vi "MultiAxisControl.vi"() -> ()   [LabVIEW 2017]
uses:
  Utility/AxisControl.ctl
  Motion/AbortSingle.vi
  Motion/MoveIncSingle.vi
  Motion/FreerunSingle.vi
  Motion/EnableSingle.vi
  Motion/DisableSingle.vi
  Motion/FaultAckSingle.vi
  Motion/HomeSingle.vi
  Parameters/GetAxisParameterString.vi
  Parameters/GetAxisParameterDouble.vi
panel:
  in  "Go":bool
  out "Status":string
  in  "StopProgram":bool caption="Stop"
  out "do stop":bool
  in  "stop":bool
  out "Error":string
  in  "Init":bool=TRUE
  in  "Abort Motion":bool
  in  "Reset Controller":bool
  in  "In Task:":i32(ring)=1 items=["Auxiliary", "T1", "T2", "T3", "T4"]
  in  "ExecuteProgram":bool caption="Execute"
  in  "Program:":path
  in  "Axes":T1[](array[typedef])
  in  "Status":string
  in  "Execute":bool
  in  "Command:":string
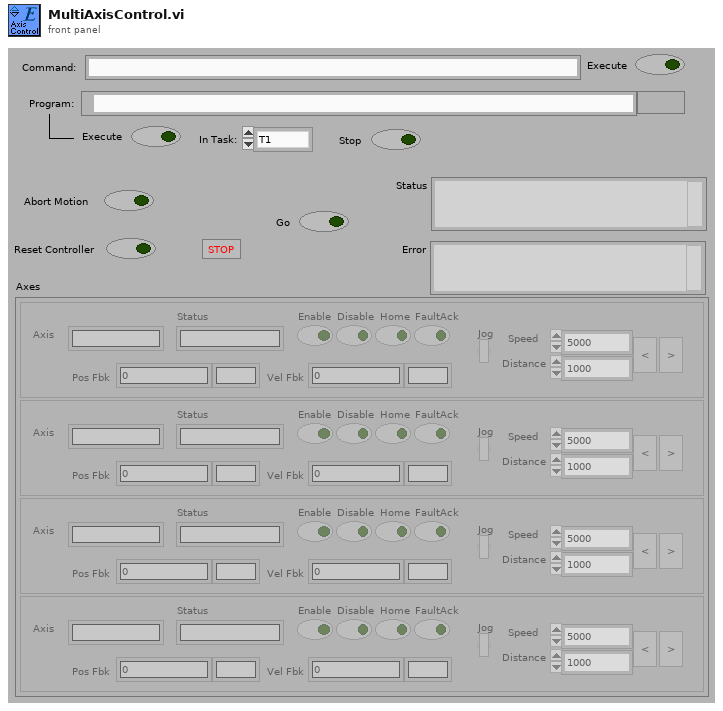
[diagram p1: front panel]
types:
  T1 = typedef "AxisControl.ctl" = cluster{"Axis":string, "Enable":bool, "Disable":bool, "Home":bool, "FaultAck":bool, "Jog":bool, "Speed":dbl, "Distance":dbl, "Jog Left":bool, "Jog Right":bool, "Status":string, "Pos Fbk":dbl, "Vel Fbk":dbl, "Pos Units":string, "Vel Units":string}
  T2 = cluster{"new reference":refnum<k24>, "Event Callback":refnum<k27>, "ControllerDiagPacket":refnum<user-event>, "Event Registration Refnum":refnum<event-registration>}
  T3 = enum32{"invalid app kind", "Development System", "Run Time System", "Student Edition", "Embedded LabVIEW", "Evaluation", "Custom"}
  T4 = cluster{"Axis":string, "Enable":bool, "Disable":bool, "Home":bool, "FaultAck":bool, "Jog":bool, "Speed":dbl, "Distance":dbl, "Jog Left":bool, "Jog Right":bool, "Status":string, "Pos Fbk":dbl, "Vel Fbk":dbl, "Pos Units":string, "Vel Units":string}
  T5 = typedef "AxisDiagPacket.ctl" = cluster{"Axis Name":string, "Acceleration Command":dbl, "Amplifier Temperature":sgl, "Analog Input 0":dbl, "Analog Input 1":dbl, "Analog Output 0":dbl, "Analog Output 1":dbl, "Axis Fault (num)":i32, "Axis Fault (str)":string, "Axis Fault (bits)":cluster{"AmplifierFault":bool, "AmplifierTemperatureFault":bool, "CcwEndOfTravelLimitFault":bool, "CcwSoftwareLimitFault":bool, "CommunicationLostFault":bool, "CwEndOfTravelLimitFault":bool, "CwSoftwareLimitFault":bool, "EmergencyStopFault":bool, "EncoderFault":bool, "ExternalFault":bool, "FeedbackScalingFault":bool, "HallSensorFault":bool, "MarkerSearchFault":bool, "MaxVelocityCommandFault":bool, "MotorTemperatureFault":bool, "None":bool, "OverCurrentFault":bool, "PositionErrorFault":bool, "PositionFeedbackFault":bool, "VelocityErrorFault":bool, "VelocityFeedbackFault":bool, "VoltageClampFault":bool, "PowerSupplyFault":bool}, "Axis Status (num)":i32, "Axis Status (str)":string, "Axis Status (bits)":cluster{"AccelerationPhase":bool, "AutofocusActive":bool, "BrakeOutput":bool, "CalibrationActive":bool, "CalibrationEnabled":bool, "CcwEndOfTravelLimitInput":bool, "CommandShapingFilterDone":bool, "CosineEncoderError":bool, "CurrentClamp":bool, "CwEndOfTravelLimitInput":bool, "DecelerationPhase":bool, "EmergencyStopInput":bool, "Enabled":bool, "GantryMasterActive":bool, "GantryModeActive":bool, "HallAInput":bool, "HallBInput":bool, "HallCInput":bool, "Homed":bool, "HomeLimitInput":bool, "Homing":bool, "InPosition":bool, "InPosition2":bool, "JoystickControl":bool, "MarkerInput":bool, "MasterMotionSuppressed":bool, "MasterSlaveControl":bool, "MotionIsCw":bool, "MoveActive":bool, "None":bool, "PositionCaptureActive":bool, "ServoControl":bool, "SineEncoderError":bool}, "Current Command":sgl, "Current Error":sgl, "Current Feedback":sgl, "Digital Input 0":i32, "Digital Input 1":i32, "Digital Input 2":i32, "Digital Output 0":i32, "Digital Output 1":i32, "Digital Output 2":i32, "Position Feedback Auxiliary":dbl, "Position Command":dbl, "Position Error":dbl, "Position Feedback":dbl, "Program Position Command":dbl, "Program Position Error":dbl, "Program Position Feedback":dbl, "Velocity Command":dbl, "Velocity Error":dbl, "Velocity Feedback":dbl}
  T6 = cluster{"Axis":string, "Enable":bool, "Disable":bool, "Home":bool, "FaultAck":bool, "Jog":bool, "Speed":dbl, "Distance":dbl, "Jog Left":bool, "Jog Right":bool, "Status":string, "Pos Fbk":dbl, "Vel Fbk":dbl, "Pos Units":string, "Vel Units":string}[]
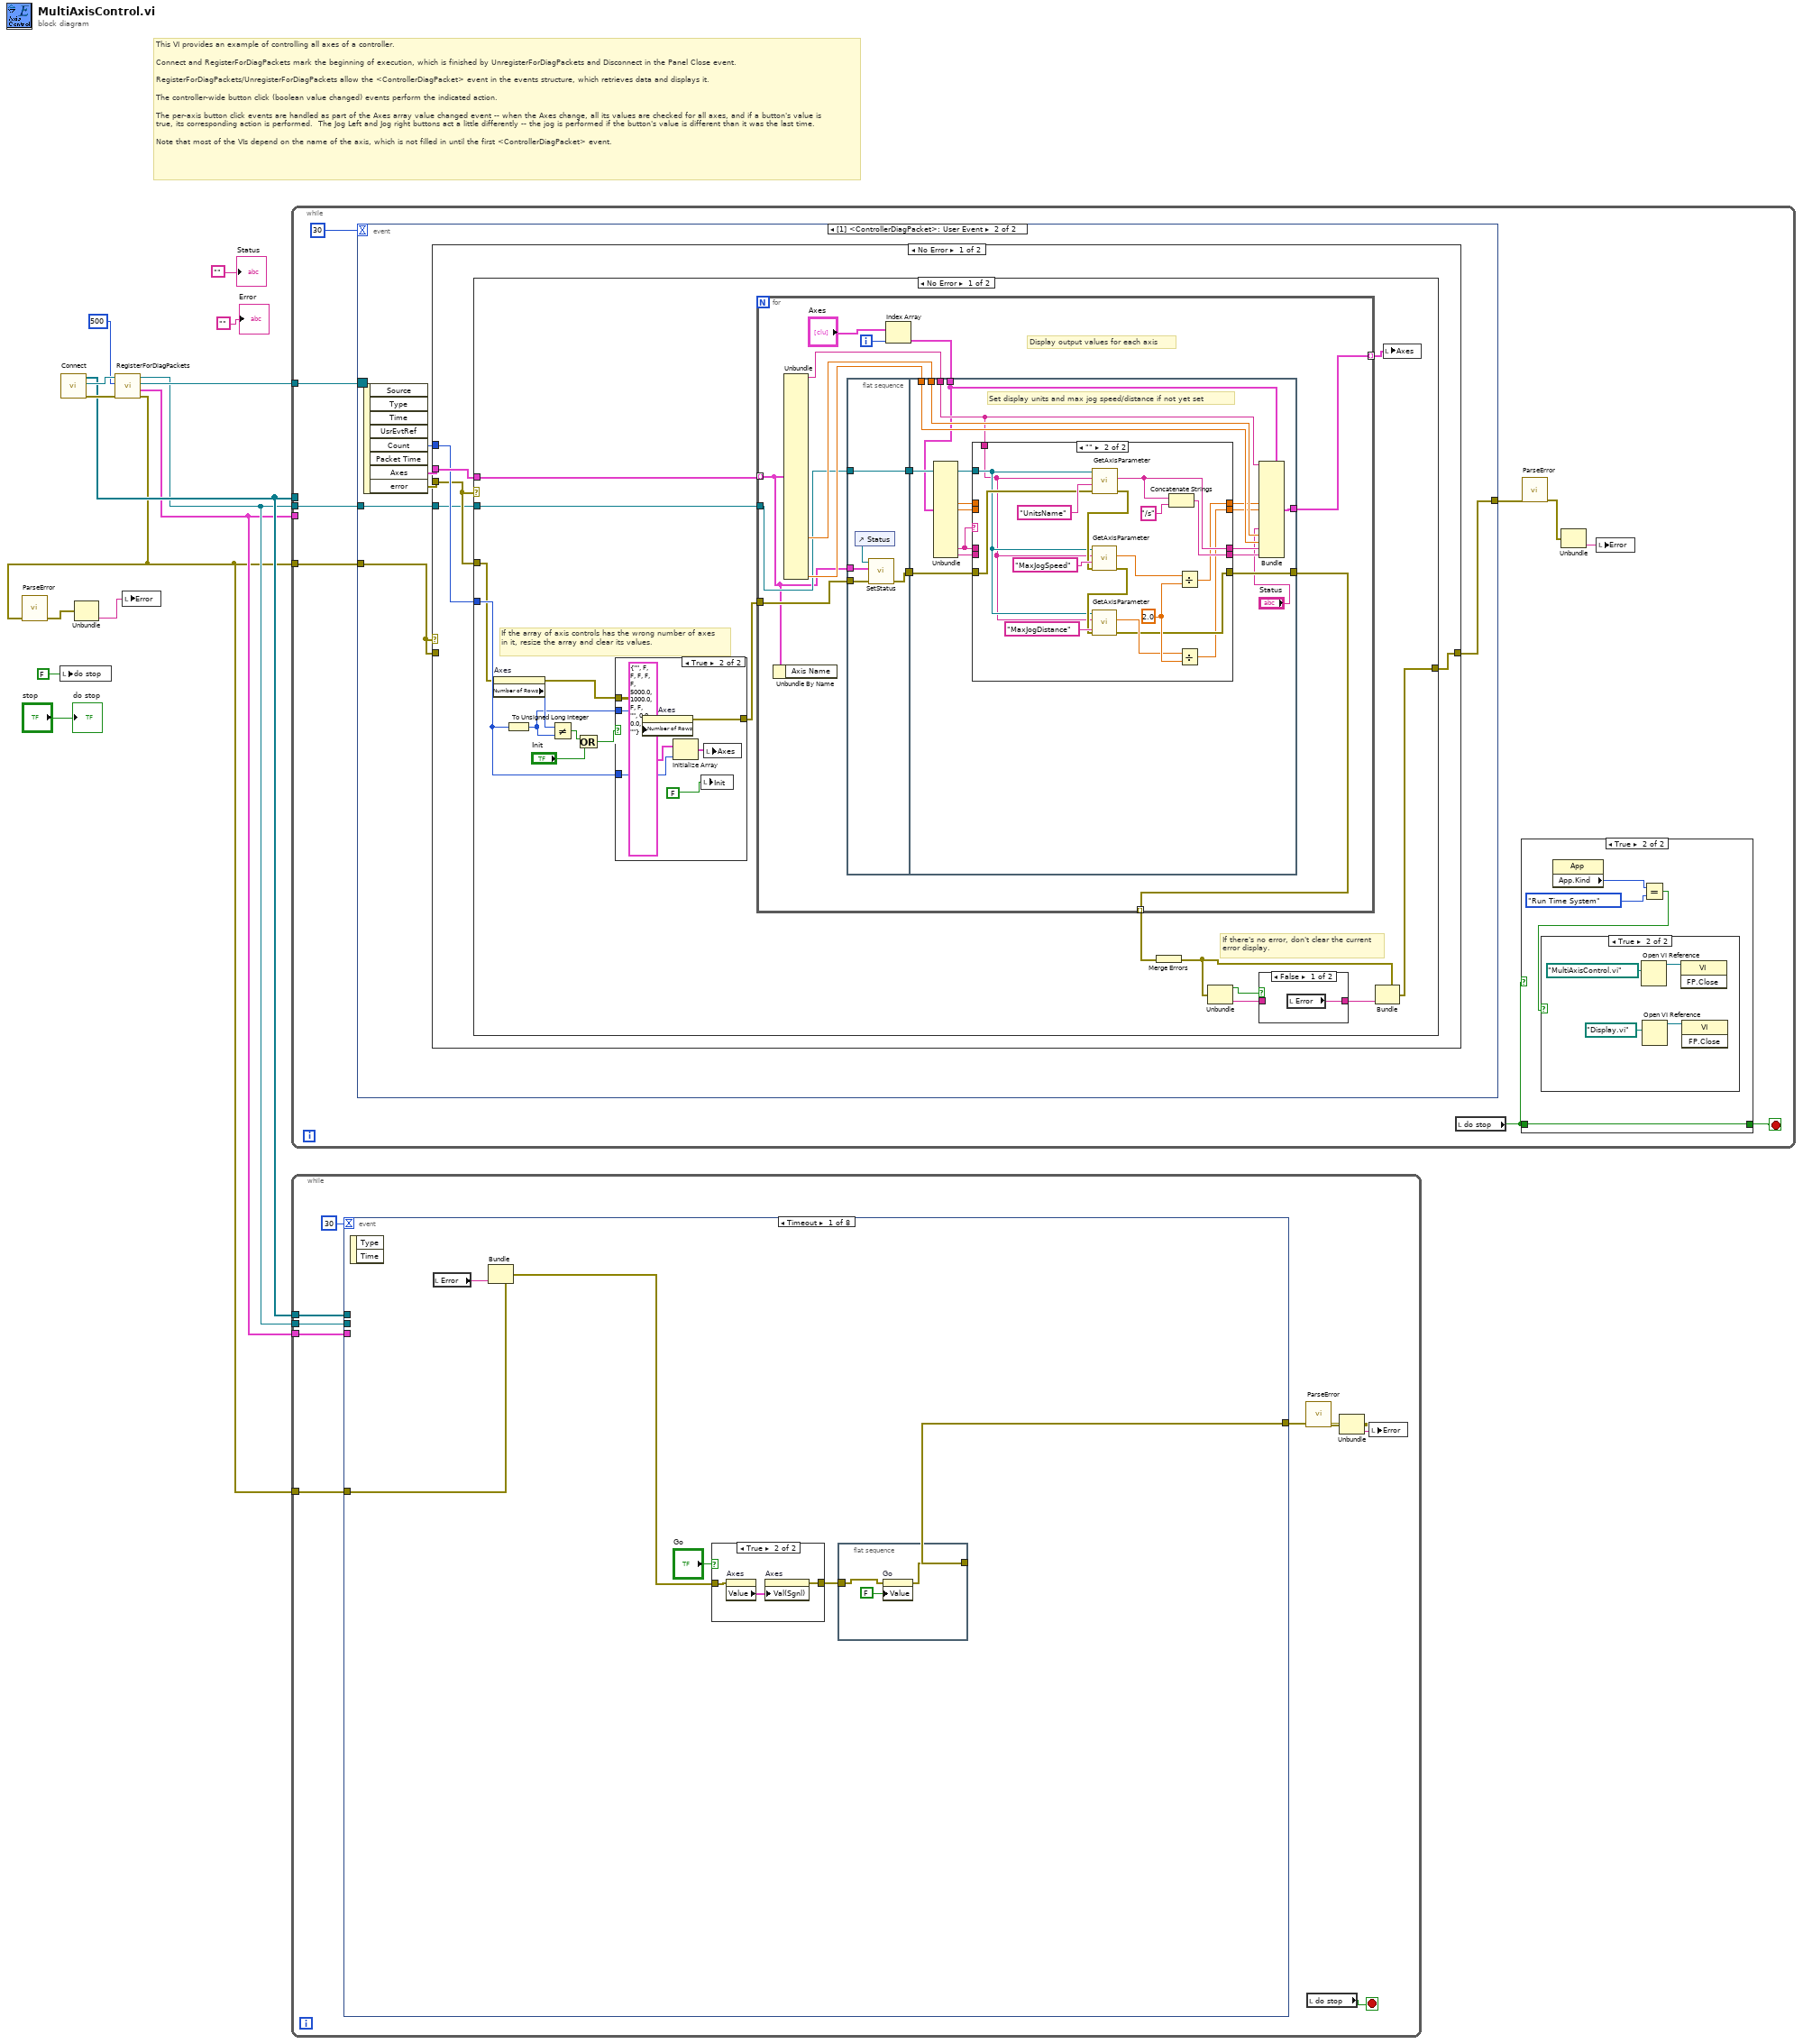
[diagram p0: block diagram]
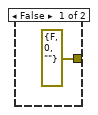
[diagram p2: hidden frame]
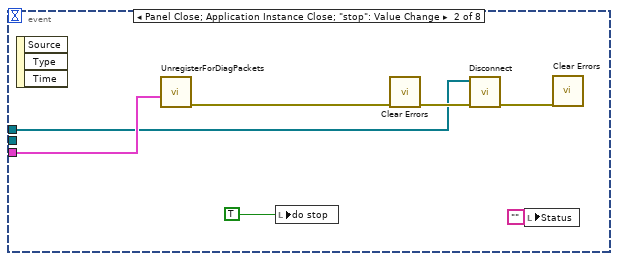
[diagram p3: hidden frame]
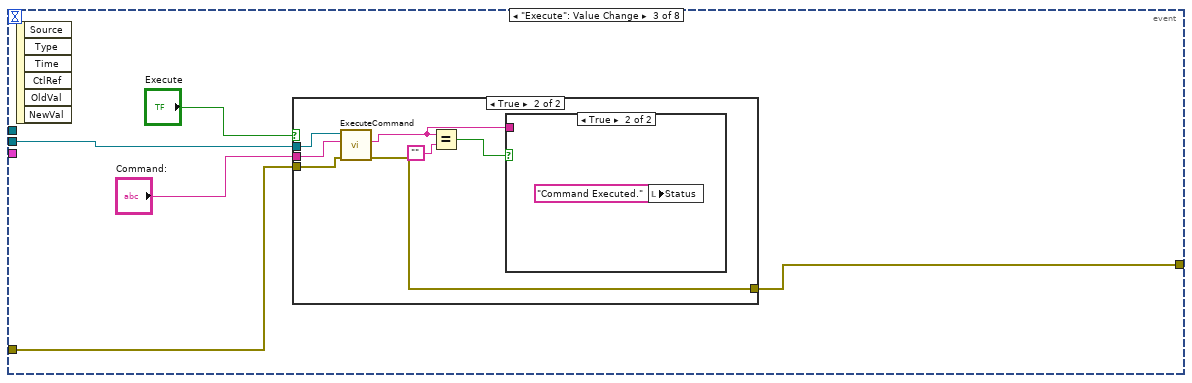
[diagram p4: hidden frame]
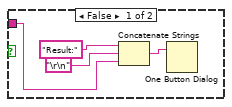
[diagram p6: hidden frame]
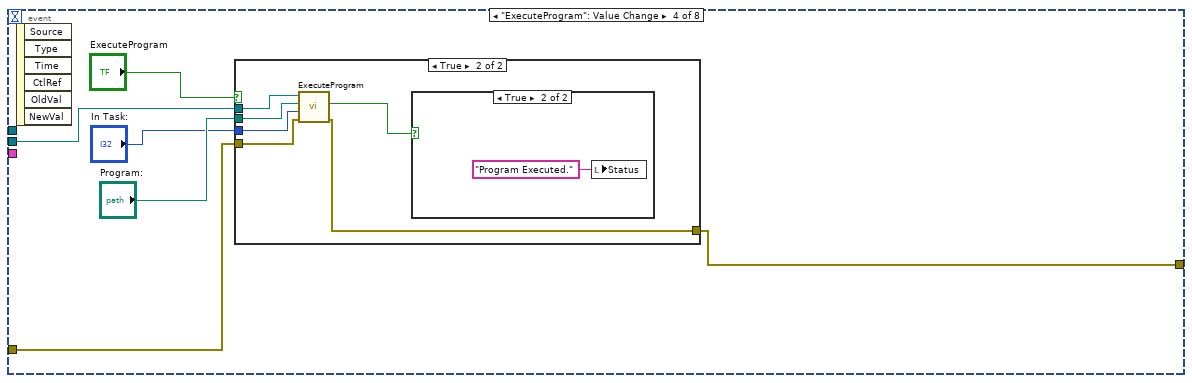
[diagram p7: hidden frame]
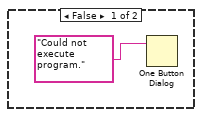
[diagram p9: hidden frame]
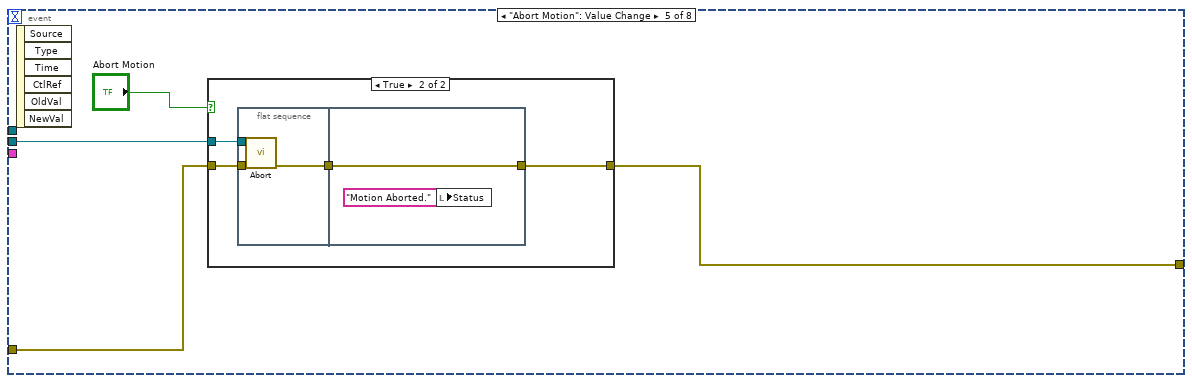
[diagram p10: hidden frame]
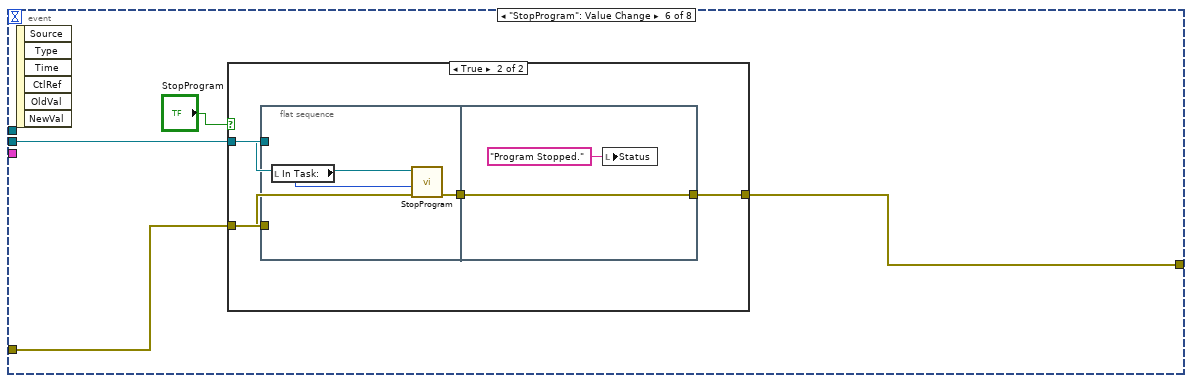
[diagram p12: hidden frame]
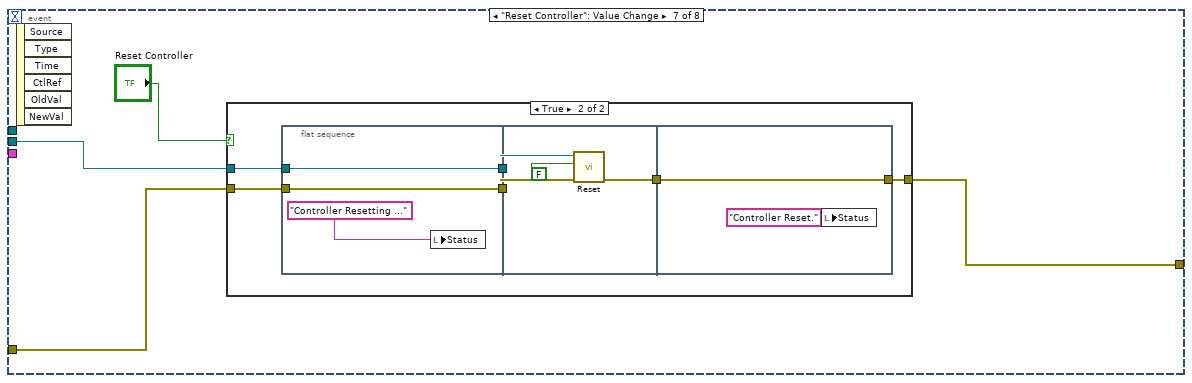
[diagram p14: hidden frame]
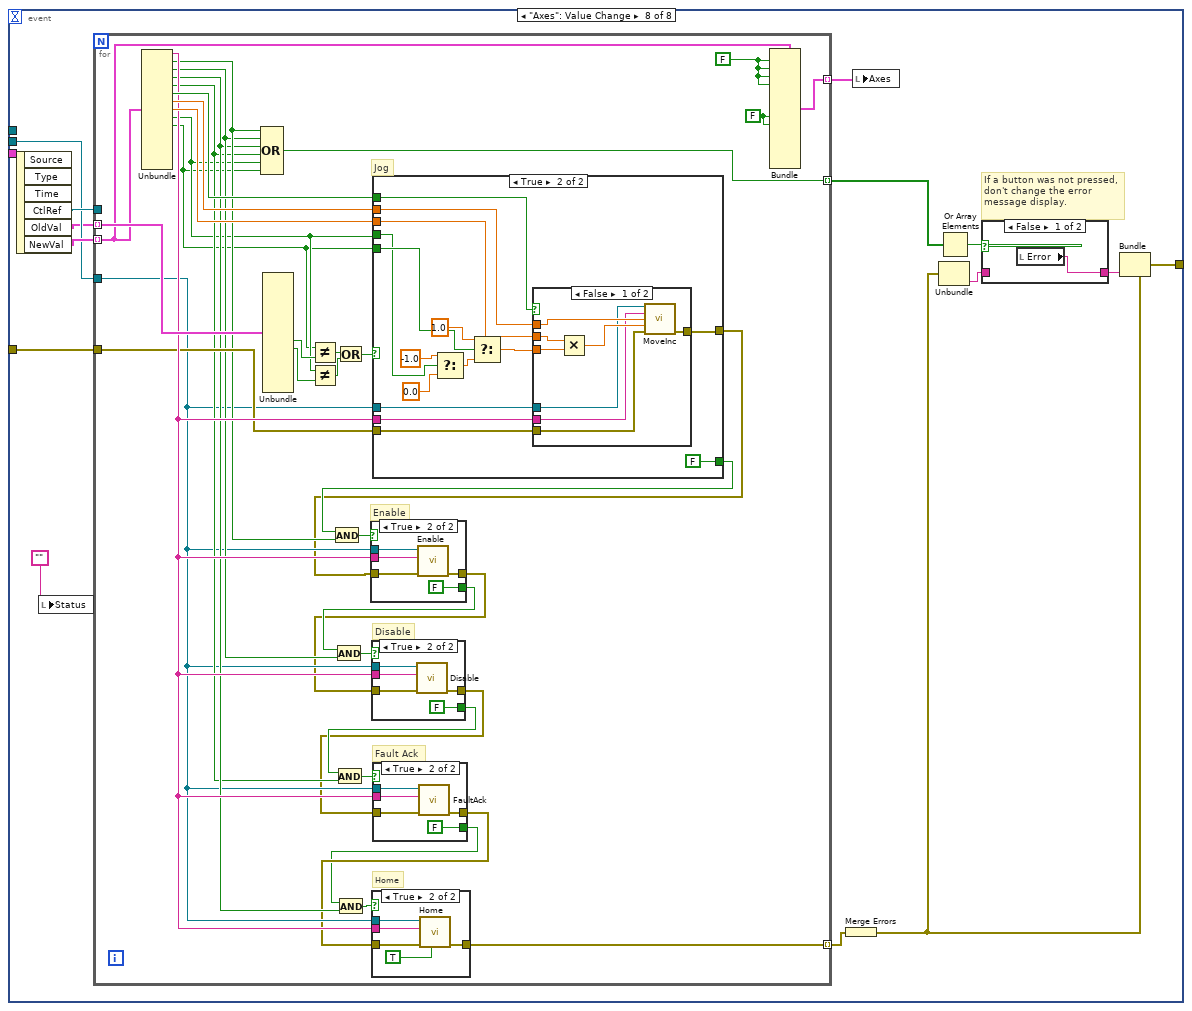
[diagram p16: hidden frame]
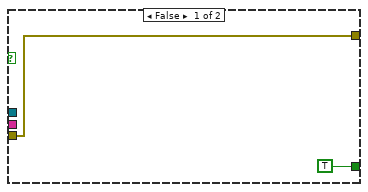
[diagram p18: hidden frame]
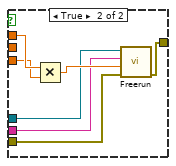
[diagram p19: hidden frame]
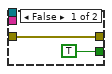
[diagram p20: hidden frame]
diagram:
  # "This VI provides an example of controlling all axes of a controller. \n\nConnect and RegisterForDiagPackets mark the beginning of execution, which is finished by UnregisterForDiagPackets and Disconnect in the Panel Close event.\n\nRegisterForDiagPackets/UnregisterForDiagPackets allow the <ControllerDiagPacket> event in the events structure, which retrieves data and displays it.\n\nThe controller-wide button click (boolean value changed) events perform the indicated action.\n\nThe per-axis button click events are handled as part of the Axes array value changed event -- when the Axes change, all its values are checked for all axes, and if a button's value is true, its corresponding action is performed.  The Jog Left and Jog right buttons act a little differently -- the jog is performed if the button's value is different than it was the last time.\n\nNote that most of the VIs depend on the name of the axis, which is not filled in until the first <ControllerDiagPacket> event."
  n1 = local write "do stop"(FALSE ("do stop")) -> ()
  n2 = call "Connect.vi"() -> ("error out"=w12:errorcluster, "controller"=w13:refnum<k24>, "controllers"=w7:refnum<k24>[])  [unwired: 9 in]
  n3 = call "RegisterForDiagPackets.vi"("error in (no error)"=w12, "refresh interval (default)"=500, "Controller in"=w13) -> ("error out"=w4:errorcluster, "Even Metadata"=w5:T2, "Event Registration Refnum"=w14:refnum<event-registration>, "Controller out"=w6:refnum<k24>)  [unwired: 4 in]
  n4 = call "ParseError.vi"("error in (no error)"=w4) -> ("error out"=w9:errorcluster)  [unwired: 10 in]
  n5 = Unbundle(w9) -> ("source"=w10:string)  [unwired: 2 out]
  n6 = local write "Error"(w10) -> ()
  n7 = while {
    tunnel: w14 -> [w20]
    tunnel: w5 -> [_]
    tunnel: w6 -> [w18]
    tunnel: w7 -> [_]
    tunnel: w4 -> [w17]
    stop <- w16 stop-if-true
    n8 = event shown="[1] <ControllerDiagPacket>: User Event" {
      selector: w20 -> [_ _]
      dyn-events: _ -> [_ _]
      timeout: 30 -> [_ _]
      tunnel: [w33 w41] -> w19
      tunnel: w18 -> [_ w40]
      tunnel: w17 -> [w35 w39]
      event Timeout {
        n9 = event-data() -> ()  [unwired: 1 in, 2 out]
        n10 = local read "Error"() -> (w34:string)
        n11 = Bundle(cluster=w35, "source"=w34) -> (w33:errorcluster)  [unwired: 2 in]
      }
      event User Event {
        n12 = event-data() -> ("Count"=w38:i32, "Axes"=w37:T5[], "error"=w36:errorcluster)  [unwired: 1 in, 5 out]
        n13 = case shown="No Error" w39 {
          tunnel: w37 -> [w46 _]
          tunnel: [w45 w133] -> w41
          tunnel: w38 -> [w44 _]
          tunnel: w36 -> [w43 _]
          tunnel: w39 -> [_ w133]
          tunnel: w40 -> [w42 _]
          frame No Error {
            n14 = case shown="No Error" w43 {
              tunnel: w46 -> [w64 _]
              tunnel: [w53 w132] -> w45
              tunnel: w43 -> [w49 w132]
              tunnel: w44 -> [w58 _]
              tunnel: w42 -> [w47 _]
              frame No Error {
                # "If there's no error, don't clear the current error display."
                # "If the array of axis controls has the wrong number of axes in it, resize the array and clear its values."
                n15 = property on="Axes" class="Arr (strict)"(error in=w49) -> (error out=w48:errorcluster, "Number of Rows"=w60:u32)  [unwired: 1 in, 1 out]
                n16 = To Unsigned Long Integer(number=w58) -> (unsigned 32bit integer=w59:u32)
                n17 = Not Equal?(x=w60, y=w59) -> (x != y?=w57:bool)
                n18 = Or(x=w57, y="Init") -> (x .or. y?=w56:bool)
                n19 = case shown="True" w56 {
                  tunnel: w48 -> [w124 w131]
                  tunnel: [w124 w130] -> w63
                  tunnel: w59 -> [_ w126]
                  tunnel: w58 -> [_ w127]
                  frame False {
                  }
                  frame True {
                    n20 = property on="Axes" class="Arr (strict)"(error in=w131, "Number of Rows"=w126) -> (error out=w130:errorcluster)  [unwired: 1 in, 1 out]
                    n21 = Initialize Array(T4 {"Axis"="", "Enable"=FALSE, "Disable"=FALSE, "Home"=FALSE, "FaultAck"=FALSE, "Jog"=FALSE, "Speed"=5000.0, "Distance"=1000.0, "Jog Left"=FALSE, "Jog Right"=FALSE, "Status"="", "Pos Fbk"=0.0, "Vel Fbk"=0.0, "Pos Units"="", "Vel Units"=""} ("Axis"), w127) -> (w129:T6)
                    n22 = local write "Init"(FALSE ("Init")) -> ()
                    n23 = local write "Axes"(w129) -> ()
                  }
                }
                n24 = for {
                  tunnel: w63 -> [w79]
                  tunnel: w64 -> [w67] mode=indexing
                  tunnel: [w78] -> w62 mode=indexing
                  tunnel: [w71] -> w61 mode=indexing
                  tunnel: w47 -> [w69]
                  i -> [w74]
                  # "Display output values for each axis"
                  n25 = Unbundle By Name(w67) -> ()  [unwired: 1 out]
                  n26 = Unbundle(w67) -> ("Axis Name"=w77:string, "Position Feedback"=w73:dbl, "Velocity Feedback"=w72:dbl)  [unwired: 29 out]
                  n27 = flat-sequence {
                    tunnel: w67 -> [w83]
                    tunnel: w79 -> [w82]
                    tunnel: [w81] -> w70
                    tunnel: w69 -> [w80]
                    tunnel: [w80] -> w68
                    tunnel: w75 -> [w94]
                    tunnel: w77 -> [w96]
                    tunnel: w73 -> [w100]
                    tunnel: w72 -> [w99]
                    tunnel: w70 -> [w97]
                    tunnel: w68 -> [w95]
                    tunnel: [w101] -> w78
                    tunnel: [w98] -> w71
                    frame #0 {
                      n28 = control-ref of="Status"() -> (w84:refnum<vi>)
                      n29 = call "SetStatus.vi"("error in (no error)"=w82, "AxisDiagPacket"=w83, "Status string"=w84) -> ("error out"=w81:errorcluster)  [unwired: 8 in]
                    }
                    frame #1 {
                      # "Set display units and max jog speed/distance if not yet set"
                      n30 = Unbundle(w94) -> ("Speed"=w89:dbl, "Distance"=w88:dbl, "Pos Units"=w93:string, "Vel Units"=w92:string)  [unwired: 11 out]
                      n31 = case shown="\"\"" w93 {
                        tunnel: w95 -> [_ w108]
                        tunnel: [w106 w111] -> w98
                        tunnel: w97 -> [w106 w121]
                        tunnel: w96 -> [_ w107]
                        tunnel: w93 -> [w104 _]
                        tunnel: w92 -> [w105 _]
                        tunnel: [w105 w120] -> w91
                        tunnel: [w104 w119] -> w90
                        tunnel: w89 -> [w103 _]
                        tunnel: w88 -> [w102 _]
                        tunnel: [w103 w110] -> w87
                        tunnel: [w102 w109] -> w86
                        frame Default {
                        }
                        frame "" {
                          w118 = 2.0 ("y")
                          n32 = call-poly "GetAxisParameter.vi"("error in (no error)"=w121, "Parameter Name"="UnitsName" ("parameter name"), "axis name"=w107, "controller in"=w108) -> ("error out"=w112:errorcluster, "value"=w119:string)  [unwired: 5 in, 1 out]
                          n33 = call-poly "GetAxisParameter.vi"("error in (no error)"=w112, "Parameter Name"="MaxJogSpeed" ("parameter name"), "axis name"=w107, "controller in"=w108) -> ("error out"=w113:errorcluster, "value"=w116:dbl)  [unwired: 5 in, 1 out]
                          n34 = call-poly "GetAxisParameter.vi"("error in (no error)"=w113, "Parameter Name"="MaxJogDistance" ("parameter name"), "axis name"=w107, "controller in"=w108) -> ("error out"=w111:errorcluster, "value"=w117:dbl)  [unwired: 5 in, 1 out]
                          n35 = Concatenate Strings(w119, "/s" ("string")) -> (w120:string)
                          n36 = Divide(x=w116, y=w118) -> (x/y=w110:dbl)
                          n37 = Divide(x=w117, y=w118) -> (x/y=w109:dbl)
                        }
                      }
                      n38 = Bundle(cluster=w94, "Axis"=w96, "Speed"=w87, "Distance"=w86, "Status"="Status", "Pos Fbk"=w100, "Vel Fbk"=w99, "Pos Units"=w90, "Vel Units"=w91) -> (w101:T1)  [unwired: 7 in]
                    }
                  }
                  n39 = Index Array(array="Axes", index=w74) -> (element=w75:T1)
                }
                n40 = Merge Errors(w61) -> (w54:errorcluster)
                n41 = Unbundle(w54) -> ("status"=w52:bool, "source"=w51:string)  [unwired: 1 out]
                n42 = case shown="False" w52 {
                  tunnel: w51 -> [_ w66]
                  tunnel: [w65 w66] -> w50
                  frame False {
                    n43 = local read "Error"() -> (w65:string)
                  }
                  frame True {
                  }
                }
                n44 = Bundle(cluster=w54, "source"=w50) -> (w53:errorcluster)  [unwired: 2 in]
                n45 = local write "Axes"(w62) -> ()
              }
              frame Error {
              }
            }
          }
          frame Error {
          }
        }
      }
    }
    n46 = local read "do stop"() -> (w15:bool)
    n47 = case shown="True" w15 {
      tunnel: w15 -> [w24 w28]
      tunnel: [w24 w28] -> w16
      frame False {
      }
      frame True {
        n48 = property class="App"() -> ("App.Kind"=w27:T3)  [unwired: 2 in, 2 out]
        n49 = Equal?(x=w27, y=T3."Run Time System" ("Application:Kind")) -> (x = y?=w25:bool)
        n50 = case shown="True" w25 {
          frame False {
          }
          frame True {
            n51 = Open VI Reference(vi path=path "MultiAxisControl.vi") -> (vi reference=w32:refnum<vi>)  [unwired: 5 in, 1 out]
            n52 = Open VI Reference(vi path=path "Display.vi") -> (vi reference=w30:refnum<vi>)  [unwired: 5 in, 1 out]
            n53 = invoke class="VI" method="FP.Close"(reference=w32) -> ()  [unwired: 2 in, 3 out]
            n54 = invoke class="VI" method="FP.Close"(reference=w30) -> ()  [unwired: 2 in, 3 out]
          }
        }
      }
    }
    n55 = call "ParseError.vi"("error in (no error)"=w19) -> ("error out"=w22:errorcluster)  [unwired: 10 in]
    n56 = Unbundle(w22) -> ("source"=w23:string)  [unwired: 2 out]
    n57 = local write "Error"(w23) -> ()
  }
  n58 = while {
    tunnel: w7 -> [w138]
    tunnel: w6 -> [w137]
    tunnel: w5 -> [w136]
    tunnel: w4 -> [w135]
    stop <- w134 stop-if-true
    n59 = event shown="[0] Timeout" {
      selector: _ -> [_ _ _ _ _ _ _ _]
      dyn-events: _ -> [_ _ _ _ _ _ _ _]
      timeout: 30 -> [_ _ _ _ _ _ _ _]
      tunnel: w136 -> [_ w162 _ _ _ _ _ _]
      tunnel: w137 -> [_ _ w166 w185 w198 w210 w227 w256]
      tunnel: w135 -> [w148 _ w165 w183 w199 w212 w226 w255]
      tunnel: [w144 _ w163 w181 w196 w211 w225 w250] -> w140
      tunnel: w138 -> [_ w159 _ _ _ _ _ _]
      event Timeout {
        n60 = event-data() -> ()  [unwired: 1 in, 2 out]
        n61 = local read "Error"() -> (w147:string)
        n62 = Bundle(cluster=w148, "source"=w147) -> (w145:errorcluster)  [unwired: 2 in]
        n63 = case shown="True" "Go" {
          tunnel: [errorcluster {"status"=FALSE, "code"=0, "source"=""} ("error out") w154] -> w143
          tunnel: w145 -> [_ w153]
          frame False {
          }
          frame True {
            n64 = property on="Axes" class="Arr (strict)"(error in=w153) -> ("Value"=w155:T1[])  [unwired: 1 in, 2 out]
            n65 = property on="Axes" class="Arr (strict)"("Val(Sgnl)"=w155) -> (error out=w154:errorcluster)  [unwired: 2 in, 1 out]
          }
        }
        n66 = flat-sequence {
          tunnel: [w150] -> w144
          tunnel: w143 -> [w149]
          frame #0 {
            n67 = property on="Go" class="Bool (strict)"(error in=w149, "Value"=FALSE ("Go")) -> (error out=w150:errorcluster)  [unwired: 1 in, 1 out]
          }
        }
      }
      event Panel Close; Application Instance Close; "stop": Value Change {
        n68 = event-data() -> ()  [unwired: 1 in, 3 out]
        n69 = call "UnregisterForDiagPackets.vi"("Even Metadata"=w162) -> ("error out"=w161:errorcluster)  [unwired: 10 in]
        n70 = local write "do stop"(TRUE) -> ()
        n71 = call <vilib>:"Clear Errors.vi"("error in (no error)"=w161) -> ("error out"=w160:errorcluster)  [unwired: 5 in, 1 out]
        n72 = call "Disconnect.vi"("error in (no error)"=w160, "controllers"=w159) -> ("error out"=w158:errorcluster)  [unwired: 9 in]
        n73 = local write "Status"("") -> ()
        n74 = call <vilib>:"Clear Errors.vi"("error in (no error)"=w158) -> ()  [unwired: 5 in, 2 out]
      }
      event "Execute": Value Change {
        n75 = event-data() -> ()  [unwired: 1 in, 6 out]
        n76 = case shown="True" "Execute" {
          tunnel: w166 -> [_ w175]
          tunnel: w165 -> [w168 w173]
          tunnel: "Command:" -> [_ w174]
          tunnel: [w168 w169] -> w163
          frame False {
          }
          frame True {
            n77 = call "ExecuteCommand.vi"("error in (no error)"=w173, "code"=w174, "controller in"=w175) -> ("error out"=w169:errorcluster, "return value"=w170:string)  [unwired: 6 in, 1 out]
            n78 = Equal?(x=w170, y="") -> (x = y?=w171:bool)
            n79 = case shown="True" w171 {
              tunnel: w170 -> [w176 _]
              frame False {
                n80 = Concatenate Strings("Result:", "\r\n", w176) -> (w179:string)
                n81 = One Button Dialog(message=w179) -> ()  [unwired: 1 in, 1 out]
              }
              frame True {
                n82 = local write "Status"("Command Executed." ("Status")) -> ()
              }
            }
          }
        }
      }
      event "ExecuteProgram": Value Change {
        n83 = event-data() -> ()  [unwired: 1 in, 6 out]
        n84 = case shown="True" "ExecuteProgram" {
          tunnel: w185 -> [_ w193]
          tunnel: w183 -> [w187 w191]
          tunnel: "Program:" -> [_ w192]
          tunnel: "In Task:" -> [_ w189]
          tunnel: [w187 w188] -> w181
          frame False {
          }
          frame True {
            n85 = call "ExecuteProgram.vi"("error in (no error)"=w191, "task id"=w189, "path"=w192, "controller in"=w193) -> ("error out"=w188:errorcluster, "success"=w190:bool)  [unwired: 5 in, 1 out]
            n86 = case shown="True" w190 {
              frame False {
                n87 = One Button Dialog(message="Could not execute program.") -> ()  [unwired: 1 in, 1 out]
              }
              frame True {
                n88 = local write "Status"("Program Executed." ("Status")) -> ()
              }
            }
          }
        }
      }
      event "Abort Motion": Value Change {
        n89 = event-data() -> ()  [unwired: 1 in, 6 out]
        n90 = case shown="True" "Abort Motion" {
          tunnel: w198 -> [_ w204]
          tunnel: w199 -> [w200 w203]
          tunnel: [w200 w202] -> w196
          frame False {
          }
          frame True {
            n91 = flat-sequence {
              tunnel: w204 -> [w207]
              tunnel: w203 -> [w206]
              tunnel: [w205] -> w201
              tunnel: [w209] -> w202
              tunnel: w201 -> [w209]
              frame #0 {
                n92 = call-poly "Abort.vi"("error in (no error)"=w206, "controller in"=w207) -> ("error out"=w205:errorcluster)  [unwired: 8 in, 1 out]
              }
              frame #1 {
                n93 = local write "Status"("Motion Aborted." ("Status")) -> ()
              }
            }
          }
        }
      }
      event "StopProgram": Value Change {
        n94 = event-data() -> ()  [unwired: 1 in, 6 out]
        n95 = case shown="True" "StopProgram" {
          tunnel: w212 -> [w214 w218]
          tunnel: [w214 w217] -> w211
          tunnel: w210 -> [_ w216]
          frame False {
          }
          frame True {
            n96 = flat-sequence {
              tunnel: w218 -> [w221]
              tunnel: w216 -> [w219]
              tunnel: [w220] -> w215
              tunnel: [w224] -> w217
              tunnel: w215 -> [w224]
              frame #0 {
                n97 = local read "In Task:"() -> (w222:i32)
                n98 = call "StopProgram.vi"("error in (no error)"=w221, "task id"=w222, "controller in"=w219) -> ("error out"=w220:errorcluster)  [unwired: 7 in, 1 out]
              }
              frame #1 {
                n99 = local write "Status"("Program Stopped." ("Status")) -> ()
              }
            }
          }
        }
      }
      event "Reset Controller": Value Change {
        n100 = event-data() -> ()  [unwired: 1 in, 6 out]
        n101 = case shown="True" "Reset Controller" {
          tunnel: w227 -> [_ w235]
          tunnel: w226 -> [w229 w234]
          tunnel: [w229 w233] -> w225
          frame False {
          }
          frame True {
            n102 = flat-sequence {
              tunnel: w234 -> [w237]
              tunnel: w235 -> [w238]
              tunnel: [w238] -> w232
              tunnel: [w237] -> w231
              tunnel: w232 -> [w242]
              tunnel: w231 -> [w241]
              tunnel: [w239] -> w230
              tunnel: [w244] -> w233
              tunnel: w230 -> [w244]
              frame #0 {
                n103 = local write "Status"("Controller Resetting ..." ("Errors")) -> ()
              }
              frame #1 {
                n104 = call "Reset.vi"("error in (no error)"=w241, "restart programs? (false)"=FALSE ("restartPrograms"), "controller in"=w242) -> ("error out"=w239:errorcluster)  [unwired: 7 in, 1 out]
              }
              frame #2 {
                n105 = local write "Status"("Controller Reset." ("Status")) -> ()
              }
            }
          }
        }
      }
      event "Axes": Value Change {
        # "If a button was not pressed, don't change the error message display."
        n106 = event-data() -> ("CtlRef"=w257:refnum<vi>, "OldVal"=w254:T1[], "NewVal"=w258:T1[])  [unwired: 1 in, 3 out]
        n107 = local write "Status"("") -> ()
        n108 = for {
          tunnel: w258 -> [w280] mode=indexing
          tunnel: w257 -> [_]
          tunnel: w256 -> [w278]
          tunnel: w255 -> [w286]
          tunnel: w254 -> [w293] mode=indexing
          tunnel: [w267] -> w253 mode=indexing
          tunnel: [w263] -> w252 mode=indexing
          tunnel: [w281] -> w247 mode=indexing
          w261 = FALSE ("Jog Left")
          w262 = FALSE
          # "Jog"
          # "Fault Ack"
          # "Home"
          # "Disable"
          # "Enable"
          n109 = Unbundle(w280) -> ("Axis"=w287:string, "Enable"=w285:bool, "Disable"=w284:bool, "Home"=w283:bool, "FaultAck"=w282:bool, "Jog"=w294:bool, "Speed"=w296:dbl, "Distance"=w295:dbl, "Jog Left"=w279:bool, "Jog Right"=w268:bool)  [unwired: 5 out]
          n110 = Compound Arithmetic op=OR(w285, w284, w283, w282, w279, w268) -> (w263:bool)
          n111 = Unbundle(w293) -> ("Jog Left"=w289:bool, "Jog Right"=w288:bool)  [unwired: 13 out]
          n112 = Not Equal?(x=w268, y=w289) -> (x != y?=w291:bool)
          n113 = Not Equal?(x=w279, y=w288) -> (x != y?=w290:bool)
          n114 = Or(x=w291, y=w290) -> (x .or. y?=w292:bool)
          n115 = case shown="True" w292 {
            tunnel: w294 -> [_ w308]
            tunnel: w296 -> [_ w306]
            tunnel: w295 -> [_ w307]
            tunnel: w268 -> [_ w302]
            tunnel: w279 -> [_ w301]
            tunnel: w278 -> [_ w305]
            tunnel: w287 -> [_ w304]
            tunnel: w286 -> [w298 w303]
            tunnel: [w298 w300] -> w271
            tunnel: [TRUE FALSE] -> w276
            frame False {
            }
            frame True {
              n116 = Select(t=-1.0, s=w301, f=0.0) -> (s? t:f=w313:dbl)
              n117 = Select(t=1.0, s=w302, f=w313) -> (s? t:f=w309:dbl)
              n118 = case shown="False" w308 {
                tunnel: w306 -> [w316 w328]
                tunnel: w307 -> [w321 _]
                tunnel: w309 -> [w320 w327]
                tunnel: w303 -> [w319 w326]
                tunnel: w304 -> [w315 w324]
                tunnel: w305 -> [w314 w323]
                tunnel: [w318 w322] -> w300
                frame False {
                  n119 = Multiply(x=w321, y=w320) -> (x*y=w317:dbl)
                  n120 = call-poly "MoveInc.vi"("controller in"=w314, "axis name"=w315, "speed"=w316, "distance"=w317, "error in (no error)"=w319) -> ("error out"=w318:errorcluster)  [unwired: 9 in, 1 out]
                }
                frame True {
                  n121 = Multiply(x=w328, y=w327) -> (x*y=w325:dbl)
                  n122 = call-poly "Freerun.vi"("error in (no error)"=w326, "speed"=w325, "axis name"=w324, "controller in"=w323) -> ("error out"=w322:errorcluster)  [unwired: 6 in, 1 out]
                }
              }
            }
          }
          n123 = And(x=w276, y=w285) -> (x .and. y?=w277:bool)
          n124 = case shown="True" w277 {
            tunnel: w278 -> [_ w355]
            tunnel: w271 -> [w350 w354]
            tunnel: w287 -> [_ w352]
            tunnel: [w350 w353] -> w270
            tunnel: [TRUE FALSE] -> w274
            frame False {
            }
            frame True {
              n125 = call-poly "Enable.vi"("error in (no error)"=w354, "axis name"=w352, "controller in"=w355) -> ("error out"=w353:errorcluster)  [unwired: 7 in, 1 out]
            }
          }
          n126 = And(x=w274, y=w284) -> (x .and. y?=w275:bool)
          n127 = case shown="True" w275 {
            tunnel: w278 -> [_ w348]
            tunnel: w270 -> [w343 w346]
            tunnel: w287 -> [_ w347]
            tunnel: [w343 w345] -> w269
            tunnel: [TRUE FALSE] -> w272
            frame False {
            }
            frame True {
              n128 = call-poly "Disable.vi"("error in (no error)"=w346, "axis name"=w347, "controller in"=w348) -> ("error out"=w345:errorcluster)  [unwired: 7 in, 1 out]
            }
          }
          n129 = And(x=w272, y=w282) -> (x .and. y?=w273:bool)
          n130 = case shown="True" w273 {
            tunnel: w278 -> [_ w335]
            tunnel: w269 -> [w330 w333]
            tunnel: w287 -> [_ w334]
            tunnel: [w330 w332] -> w266
            tunnel: [TRUE FALSE] -> w264
            frame False {
            }
            frame True {
              n131 = call-poly "FaultAck.vi"("error in (no error)"=w333, "axis name"=w334, "controller in"=w335) -> ("error out"=w332:errorcluster)  [unwired: 7 in, 1 out]
            }
          }
          n132 = And(x=w264, y=w283) -> (x .and. y?=w265:bool)
          n133 = case shown="True" w265 {
            tunnel: w278 -> [_ w341]
            tunnel: w287 -> [_ w340]
            tunnel: w266 -> [w336 w339]
            tunnel: [w336 w338] -> w267
            frame False {
            }
            frame True {
              n134 = call-poly "Home.vi"("return immediately"=TRUE ("Return Immediately ?"), "error in (no error)"=w339, "axis name"=w340, "controller in"=w341) -> ("error out"=w338:errorcluster)  [unwired: 6 in, 1 out]
            }
          }
          n135 = Bundle(cluster=w280, "Enable"=w262, "Disable"=w262, "Home"=w262, "FaultAck"=w262, "Jog Left"=w261, "Jog Right"=w261) -> (w281:T1)  [unwired: 9 in]
        }
        n136 = Merge Errors(w253) -> (w246:errorcluster)
        n137 = local write "Axes"(w247) -> ()
        n138 = Unbundle(w246) -> ("source"=w249:string)  [unwired: 2 out]
        n139 = Or Array Elements(Boolean array=w252) -> (logical OR=w251:bool)
        n140 = case shown="False" w251 {
          tunnel: w249 -> [_ w260]
          tunnel: [w259 w260] -> w248
          frame False {
            n141 = local read "Error"() -> (w259:string)
          }
          frame True {
          }
        }
        n142 = Bundle(cluster=w246, "source"=w248) -> (w250:errorcluster)  [unwired: 2 in]
      }
    }
    n143 = call "ParseError.vi"("error in (no error)"=w140) -> ("error out"=w142:errorcluster)  [unwired: 10 in]
    n144 = local read "do stop"() -> (w134:bool)
    n145 = Unbundle(w142) -> ("source"=w141:string)  [unwired: 2 out]
    n146 = local write "Error"(w141) -> ()
  }
  "Error" <- ""
  "do stop" <- "stop"
  "Status" <- ""
